vi "Emballage_BDD_lecture_EMBALLAGE_PARAM_join.vi"(8 "error in":errorcluster) -> (0 "error out":errorcluster, 1 "données":string[][](array[string]), 2 "Colonne":string[](array[string])=["ID_ARTICLE_GPAO", "NOVALVE_FILTRE", "INDICE_PRODUIT", "AFFICHE_CODEBARRE_CLIENT", "MELANGE_LOT_POSSIBLE", "FAMILLE_VALVE", "REMARQUE"], 3 "tableauHeaders":string[][](array[string]))   [LabVIEW 2020]
uses:
  Modules/FS/60_FS_Controles/60_FS_SetGet.ctl
  <vilib>/addons/database/Connection.llb/DB Tools Open Connec (Path).vi
  <vilib>/addons/database/Connection.llb/Conn Execute.vi
  <vilib>/addons/database/Recordset.llb/Rec Fetch Recordset Data (R).vi
  <vilib>/addons/database/Recordset.llb/Rec Destroy - Connection.vi
  <vilib>/addons/database/NI_Database_API.lvlib
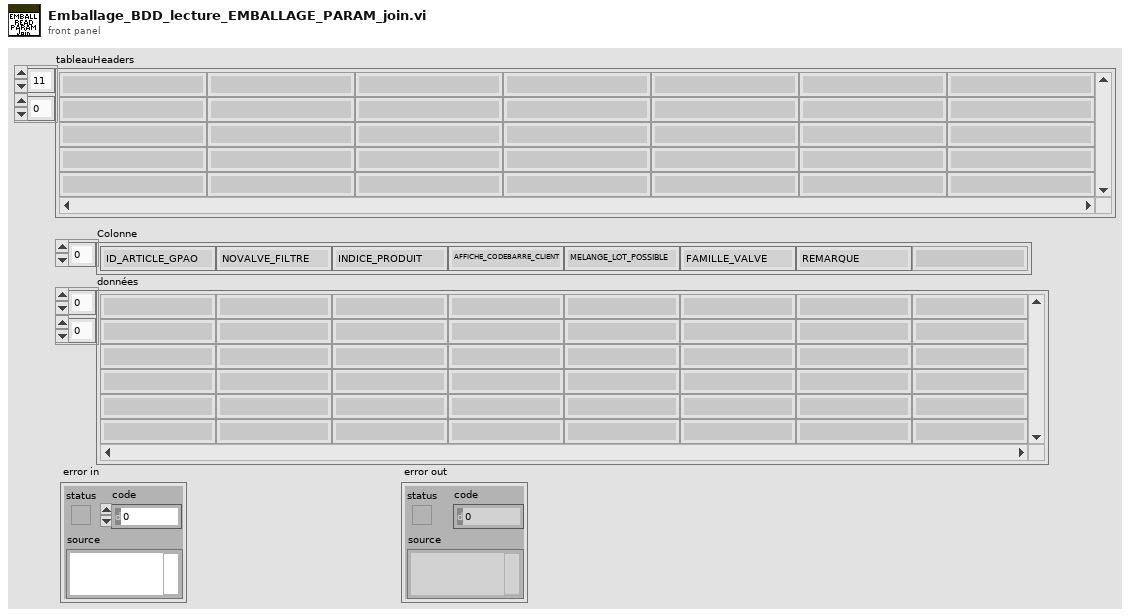
[diagram p1: front panel]
types:
  T1 = typedef "60_FS_SetGet.ctl" = enum16{"set", "get"}
  T2 = typedef "60_FS_CLT_Chemins.ctl" = cluster{"Racine_local":path, "Racine_reseau":path, "Racine_Support_Application":path, "Fichier_Journalisation":path, "Connexion_BDD_VSX":path, "Connexion_BDD_PLZ":path}
  T3 = typedef "NI_Database_API.lvlib/Conn ObjectReference.ctl" = refnum<k1>
  T4 = typedef "NI_Database_API.lvlib/Rec ObjectReference.ctl" = refnum<k1>
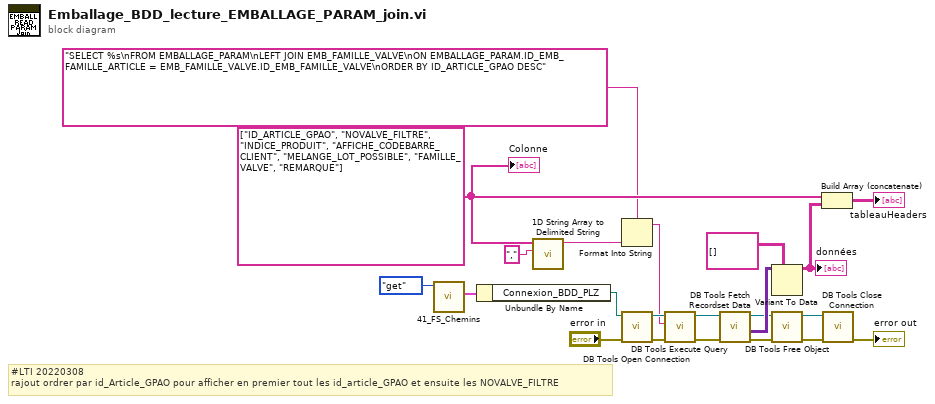
[diagram p0: block diagram]
diagram:
  w5 = string[] ["ID_ARTICLE_GPAO", "NOVALVE_FILTRE", "INDICE_PRODUIT", "AFFICHE_CODEBARRE_CLIENT", "MELANGE_LOT_POSSIBLE", "FAMILLE_VALVE", "REMARQUE"]
  # "#LTI 20220308\nrajout ordrer par id_Article_GPAO pour afficher en premier tout les id_article_GPAO et ensuite les NOVALVE_FILTRE"
  n1 = call "41_FS_Chemins.vi"("SetGet"=60_FS_SetGet."get") -> ("CLT_Chemins_out"=w7:T2)  [unwired: 9 in, 1 out]
  n2 = Unbundle By Name(w7) -> ("Connexion_BDD_PLZ"=w6:path)
  n3 = call <vilib>:"1D String Array to Delimited String.vi"("delimiter"=",", "string array"=w5) -> ("delimited string"=w1:string)  [unwired: 9 in]
  n4 = Format Into String(format string="SELECT %s\nFROM EMBALLAGE_PARAM\nLEFT JOIN EMB_FAMILLE_VALVE\nON EMBALLAGE_PARAM.ID_EMB_FAMILLE_ARTICLE = EMB_FAMILLE_VALVE.ID_EMB_FAMILLE_VALVE\nORDER BY ID_ARTICLE_GPAO DESC" ("SQL query"), w1) -> (resulting string=w3:string)  [unwired: 2 in, 1 out]
  n5 = call-poly <vilib>:"DB Tools Open Connection.vi"("error in (no error)"="error in", "connection information"=w6) -> ("error out"=w11:errorcluster, "connection reference"=w12:T3)  [unwired: 6 in]
  n6 = call-poly <vilib>:"DB Tools Execute Query.vi"("error in (no error)"=w11, "SQL query"=w3, "connection reference"=w12) -> ("error out"=w21:errorcluster, "recordset reference"=w13:T4)  [unwired: 5 in]
  n7 = call-poly <vilib>:"DB Tools Fetch Recordset Data.vi"("error in (no error)"=w21, "recordset reference"=w13) -> ("error out"=w16:errorcluster, "recordset data"=w20:variant[][], "recordset reference out"=w17:T4)  [unwired: 3 in]
  n8 = Variant To Data(type=string[][] [] ("Liste des champs à lire 2"), Variant=w20) -> (data=w10:string[][])  [unwired: 1 in, 1 out]
  "données" <- w10
  n9 = call-poly <vilib>:"DB Tools Free Object.vi"("error in (no error)"=w16, "recordset reference"=w17) -> ("error out"=w15:errorcluster, "connection reference"=w14:T3)  [unwired: 8 in]
  n10 = Build Array (concatenate)(w5, w10) -> (→"tableauHeaders":string[][])
  n11 = call <vilib>:"DB Tools Close Connection.vi"("error in (no error)"=w15, "connection reference"=w14) -> ("error out"=→"error out":errorcluster)  [unwired: 5 in]
  "Colonne" <- w5
